vi "quiz3.3.vi"() -> ()   [LabVIEW 2017]
panel:
  out "Tab Control 2":enum32{"Login", "Menu", "Add", "delete"}(tab)
  in  "Ingresar 2":bool
  in  "Contraseña 2":string
  in  "Usuario 2":string
  in  "Delete Button 2":bool
  in  "Add Button 2":bool
  in  "Home Button 2":bool
  out "Cusuario 2":string
  in  "Previous Button 3":bool
  in  "AddContraseña 2":string
  in  "AddUsuario 2":string
  in  "Agregar 2":bool
  out "Agregado 2":bool
  in  "Cancel Button 2":bool
  in  "DeleteUsuario 3":string
  in  "Previous Button 4":bool
  out "text 2":string
  out "Tab Control":enum32{"Login", "Menu", "Add", "delete"}(tab)
  in  "Ingresar":bool
  in  "Contraseña":string
  in  "Usuario":string
  in  "Delete Button":bool
  in  "Add Button":bool
  in  "Home Button":bool
  out "Cusuario":string
  in  "Previous Button":bool
  in  "AddContraseña":string
  in  "AddUsuario":string
  in  "Agregar":bool
  out "Agregado":bool
  in  "Cancel Button":bool
  in  "DeleteUsuario":string
  in  "Previous Button 2":bool
  out "text":string
  # "USTED INGRESO CON EL USUARIO"
  # "USTED INGRESO CON EL USUARIO"
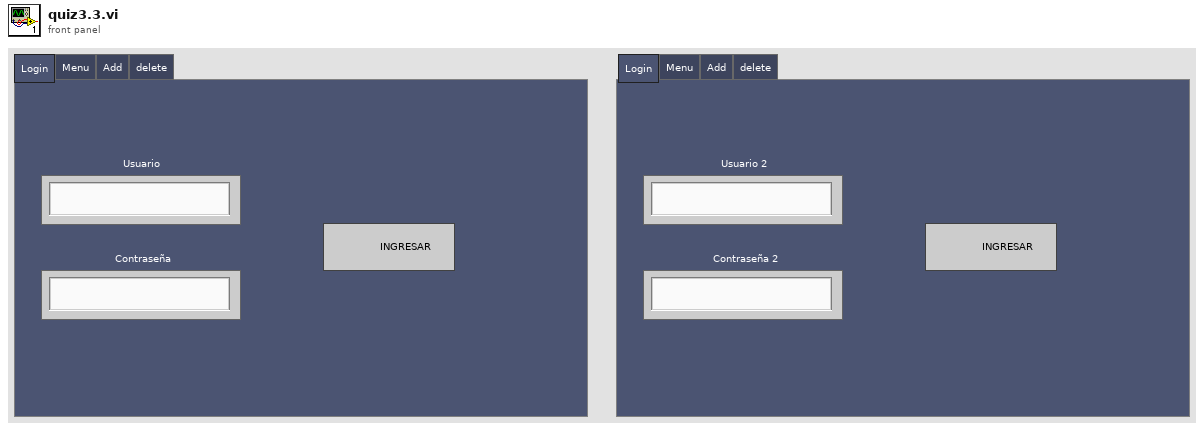
[diagram p1: front panel]
types:
  T1 = enum16{"open", "replace", "create", "open or create", "replace or create", "replace or create with confirmation"}
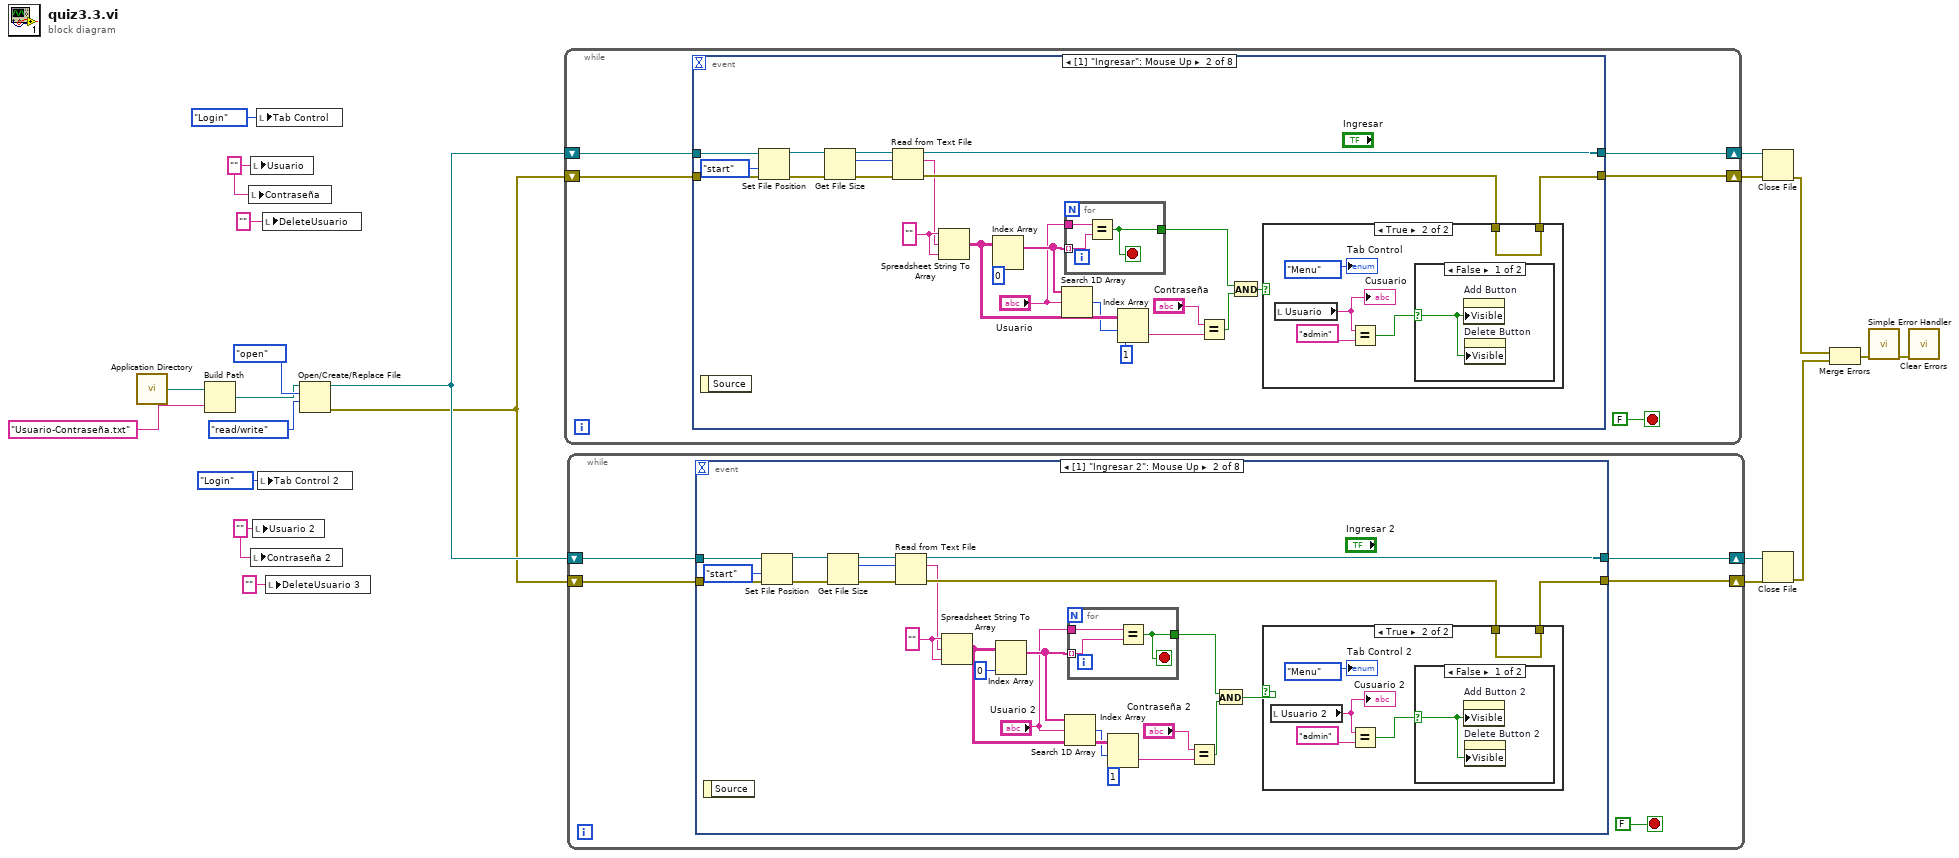
[diagram p0: block diagram]
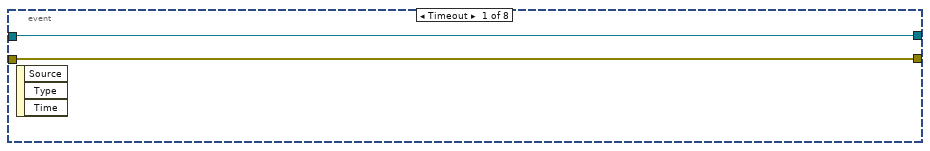
[diagram p2: hidden frame]
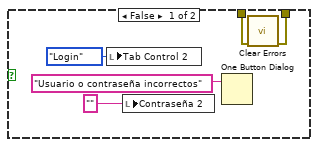
[diagram p3: hidden frame]
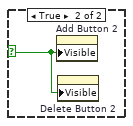
[diagram p4: hidden frame]
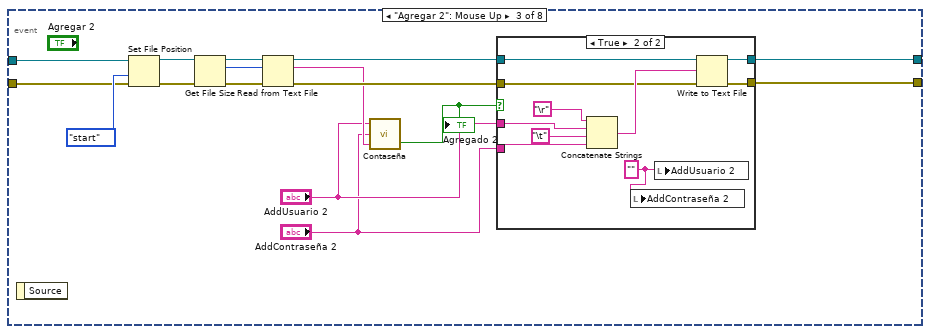
[diagram p5: hidden frame]
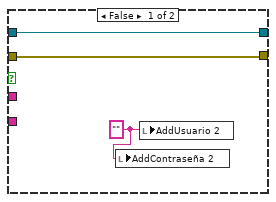
[diagram p6: hidden frame]
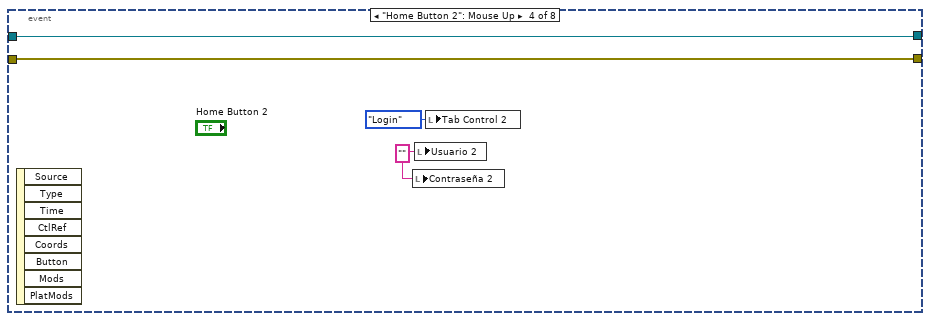
[diagram p7: hidden frame]
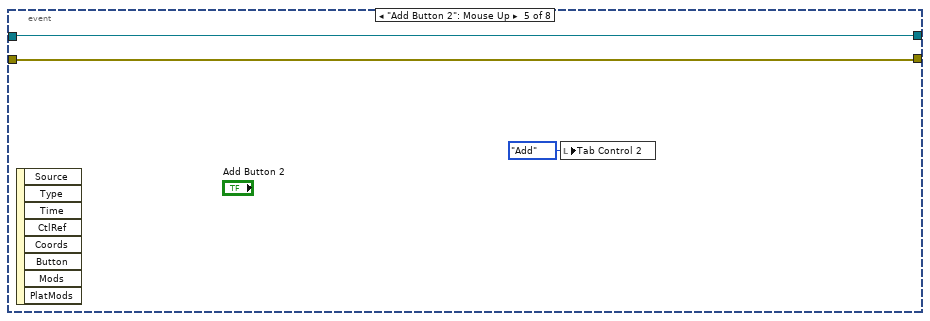
[diagram p8: hidden frame]
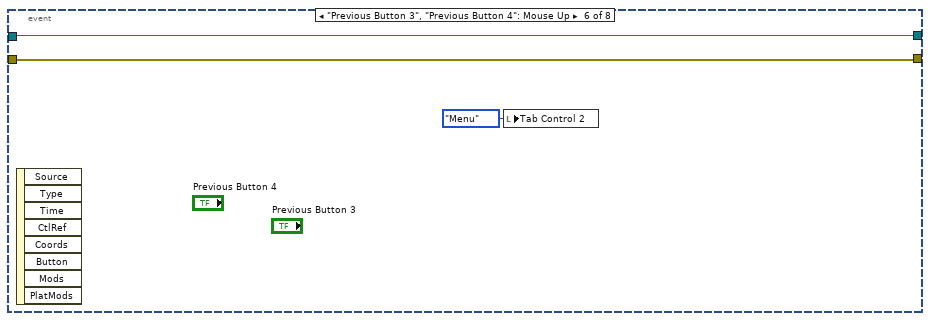
[diagram p9: hidden frame]
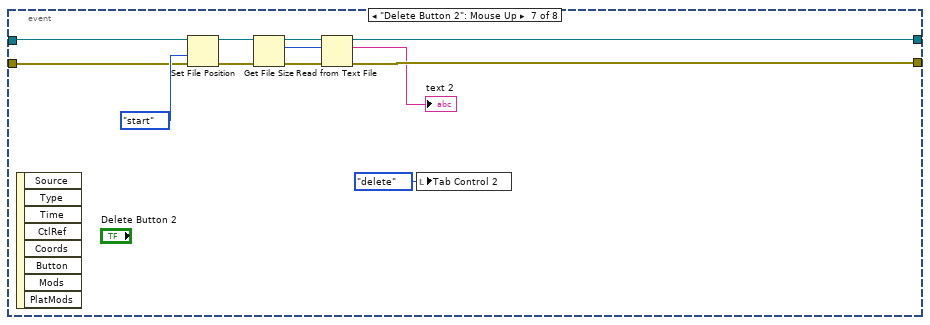
[diagram p10: hidden frame]
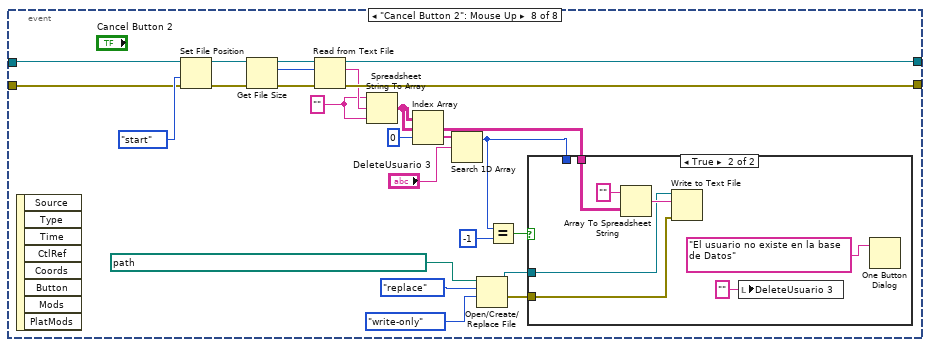
[diagram p11: hidden frame]
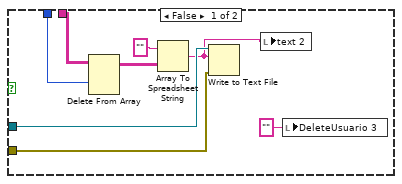
[diagram p12: hidden frame]
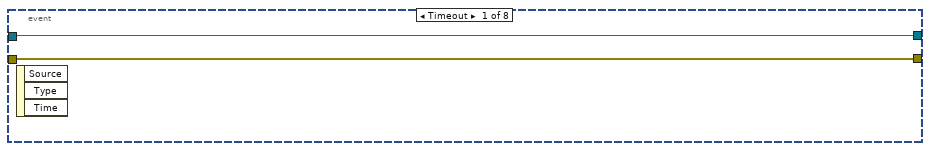
[diagram p13: hidden frame]
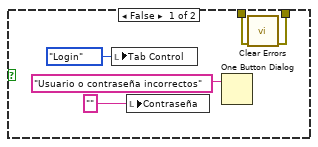
[diagram p14: hidden frame]
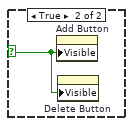
[diagram p15: hidden frame]
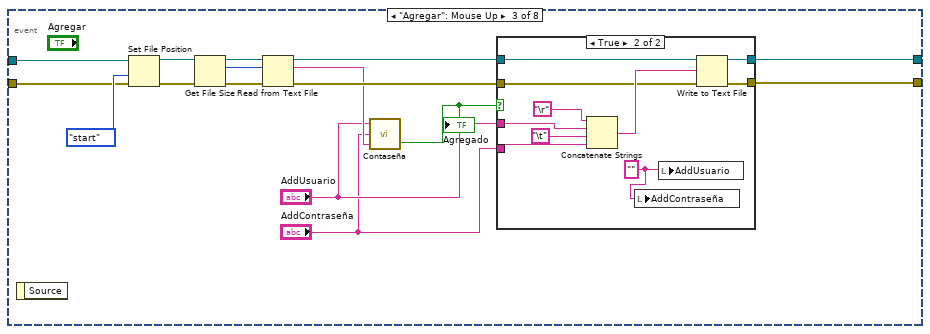
[diagram p16: hidden frame]
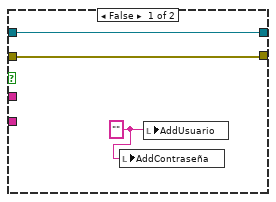
[diagram p17: hidden frame]
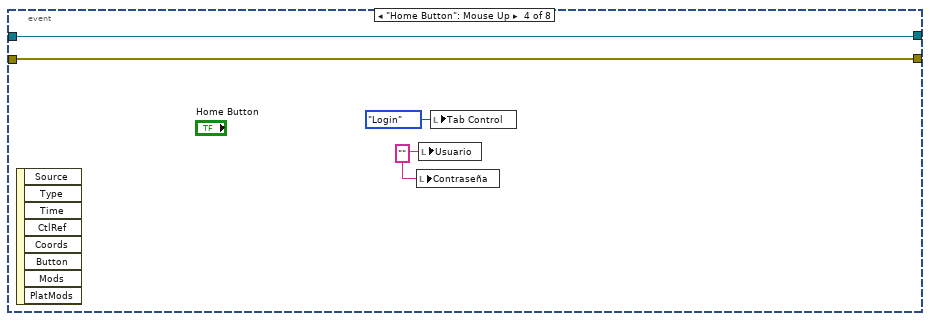
[diagram p18: hidden frame]
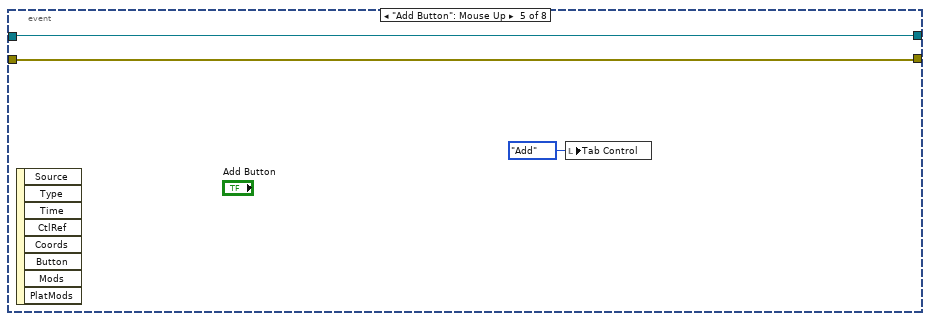
[diagram p19: hidden frame]
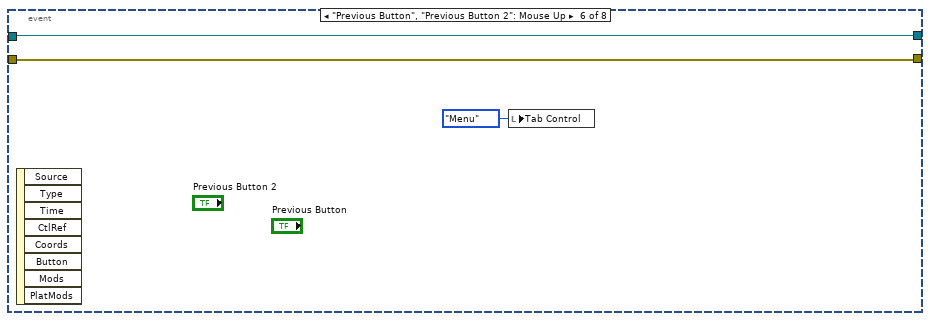
[diagram p20: hidden frame]
diagram:
  w1 = "" ("Usuario")
  w14 = "" ("Usuario")
  n1 = call <vilib>:"Application Directory.vi"() -> ("Application Directory"=w21:path)
  n2 = Build Path(base path=w21, name or relative path="Usuario-Contraseña.txt") -> (appended path=w15:path)
  n3 = local write "Contraseña"(w14) -> ()
  n4 = local write "Usuario"(w14) -> ()
  n5 = local write "Contraseña 2"(w1) -> ()
  n6 = local write "Usuario 2"(w1) -> ()
  n7 = local write "Tab Control"(enum32{"Login", "Menu", "Add", "delete"}."Login" ("Tab Control")) -> ()
  n8 = local write "Tab Control 2"(enum32{"Login", "Menu", "Add", "delete"}."Login" ("Tab Control")) -> ()
  n9 = local write "DeleteUsuario"("" ("DeleteUsuario 2")) -> ()
  n10 = local write "DeleteUsuario 3"("" ("DeleteUsuario 2")) -> ()
  n11 = Open/Create/Replace File(file path (use dialog)=w15, operation (0:open)=T1."open", access (0:read/write)=enum16{"read/write", "read-only", "write-only"}."read/write") -> (refnum out=w5:refnum<file>, error out=w4:errorcluster)  [unwired: 3 in, 1 out]
  n12 = while {
    shift-right: [w23] -> w11
    shift-left: w5 -> [w24]
    shift-right: [w22] -> w16
    shift-left: w4 -> [w25]
    stop <- FALSE stop-if-true
    n13 = event shown="[1] \"Ingresar\": Mouse Up" {
      selector: _ -> [_ _ _ _ _ _ _ _]
      dyn-events: _ -> [_ _ _ _ _ _ _ _]
      timeout: _ -> [_ _ _ _ _ _ _ _]
      tunnel: w25 -> [w27 w52 w71 w98 w102 w105 w109 w136]
      tunnel: [w28 w47 w83 w99 w103 w106 w110 w132] -> w23
      tunnel: [w27 w44 w82 w98 w102 w105 w108 w131] -> w22
      tunnel: w24 -> [w28 w46 w72 w99 w103 w106 w111 w135]
      event Timeout {
        n14 = event-data() -> ()  [unwired: 1 in, 3 out]
      }
      event "Ingresar": Mouse Up {
        w40 = "" ("format string")
        n15 = event-data() -> ()  [unwired: 1 in, 1 out]
        n16 = Set File Position(refnum=w46, from (0:start)=enum16{"start", "end", "current"}."start", error in=w52) -> (refnum out=w50:refnum<file>, error out=w51:errorcluster)  [unwired: 1 in]
        n17 = Get File Size(file=w50, error in=w51) -> (refnum out=w42:refnum<file>, size (in bytes)=w49:i64, 0:w48:errorcluster)
        n18 = Read from Text File(file (use dialog)=w42, count=w49, error in=w48) -> (refnum out=w47:refnum<file>, text=w39:string, error out=w45:errorcluster)  [unwired: 1 in, 1 out]
        n19 = Spreadsheet String To Array(format string=w40, spreadsheet string=w39, array type (2D Dbl)=w40) -> (array=w35:string[][])  [unwired: 1 in]
        n20 = Index Array(array=w35, index (col)=0 ("index")) -> (element=w37:string[])  [unwired: 1 in]
        n21 = Search 1D Array(1D array=w37, element="Usuario") -> (index of element=w32:i32)  [unwired: 1 in]
        n22 = for {
          tunnel: "Usuario" -> [w55]
          tunnel: [w54] -> w38
          tunnel: w37 -> [w53] mode=indexing
          stop <- w54 stop-if-true
          n23 = Equal?(x=w55, y=w53) -> (x = y?=w54:bool)
        }
        n24 = Index Array(array=w35, index (row)=w32, index (col)=1 ("index")) -> (element=w30:string)
        n25 = Equal?(x="Contraseña", y=w30) -> (x = y?=w34:bool)
        n26 = And(x=w38, y=w34) -> (x .and. y?=w41:bool)
        n27 = case shown="True" w41 {
          tunnel: [w58 w65] -> w44
          tunnel: w45 -> [w57 w65]
          frame False {
            n28 = local write "Tab Control"(enum32{"Login", "Menu", "Add", "delete"}."Login" ("Tab Control")) -> ()
            n29 = local write "Contraseña"("" ("Usuario")) -> ()
            n30 = One Button Dialog(message="Usuario o contraseña incorrectos") -> ()  [unwired: 1 in, 1 out]
            n31 = call <vilib>:"Clear Errors.vi"("error in (no error)"=w57) -> ("error out"=w58:errorcluster)  [unwired: 5 in, 1 out]
          }
          frame True {
            n32 = local read "Usuario"() -> (w63:string)
            "Cusuario" <- w63
            n33 = Equal?(x=w63, y="admin") -> (x = y?=w64:bool)
            n34 = case shown="False" w64 {
              selector: w64 -> [w66 w67]
              frame False {
                n35 = property on="Add Button" class="Bool (strict)"("Visible"=w66) -> ()  [unwired: 2 in, 2 out]
                n36 = property on="Delete Button" class="Bool (strict)"("Visible"=w66) -> ()  [unwired: 2 in, 2 out]
              }
              frame True {
                n37 = property on="Add Button" class="Bool (strict)"("Visible"=w67) -> ()  [unwired: 2 in, 2 out]
                n38 = property on="Delete Button" class="Bool (strict)"("Visible"=w67) -> ()  [unwired: 2 in, 2 out]
              }
            }
            "Tab Control" <- enum32{"Login", "Menu", "Add", "delete"}."Menu" ("Tab Control")
          }
        }
      }
      event "Agregar": Mouse Up {
        n39 = event-data() -> ()  [unwired: 1 in, 1 out]
        n40 = Set File Position(refnum=w72, from (0:start)=enum16{"start", "end", "current"}."start", error in=w71) -> (refnum out=w79:refnum<file>, error out=w80:errorcluster)  [unwired: 1 in]
        n41 = Get File Size(file=w79, error in=w80) -> (refnum out=w76:refnum<file>, size (in bytes)=w78:i64, 0:w77:errorcluster)
        n42 = Read from Text File(file (use dialog)=w76, count=w78, error in=w77) -> (refnum out=w74:refnum<file>, text=w70:string, error out=w73:errorcluster)  [unwired: 1 in, 1 out]
        n43 = call "Contaseña.vi"("spreadsheet string"=w70, "AddContraseña"="AddContraseña", "addUsuario"="AddUsuario") -> ("result"=w81:bool)  [unwired: 1 out]
        "Agregado" <- w81
        n44 = case shown="True" w81 {
          tunnel: [w86 w96] -> w83
          tunnel: [w85 w95] -> w82
          tunnel: w74 -> [w86 w91]
          tunnel: w73 -> [w85 w90]
          tunnel: "AddUsuario" -> [_ w89]
          tunnel: "AddContraseña" -> [_ w88]
          frame False {
            w84 = "" ("Usuario")
            n45 = local write "AddContraseña"(w84) -> ()
            n46 = local write "AddUsuario"(w84) -> ()
          }
          frame True {
            w87 = "" ("Usuario")
            n47 = Concatenate Strings("\r", w89, "\t", w88) -> (w94:string)
            n48 = local write "AddContraseña"(w87) -> ()
            n49 = local write "AddUsuario"(w87) -> ()
            n50 = Write to Text File(file (use dialog)=w91, text=w94, error in=w90) -> (refnum out=w96:refnum<file>, error out=w95:errorcluster)  [unwired: 1 in, 1 out]
          }
        }
      }
      event "Home Button": Mouse Up {
        w100 = "" ("Usuario")
        n51 = event-data() -> ()  [unwired: 1 in, 8 out]
        n52 = local write "Contraseña"(w100) -> ()
        n53 = local write "Usuario"(w100) -> ()
        n54 = local write "Tab Control"(enum32{"Login", "Menu", "Add", "delete"}."Login" ("Tab Control")) -> ()
      }
      event "Add Button": Mouse Up {
        n55 = event-data() -> ()  [unwired: 1 in, 8 out]
        n56 = local write "Tab Control"(enum32{"Login", "Menu", "Add", "delete"}."Add" ("Tab Control")) -> ()
      }
      event "Previous Button", "Previous Button 2": Mouse Up {
        n57 = event-data() -> ()  [unwired: 1 in, 8 out]
        n58 = local write "Tab Control"(enum32{"Login", "Menu", "Add", "delete"}."Menu" ("Tab Control")) -> ()
      }
      event "Delete Button": Mouse Up {
        n59 = event-data() -> ()  [unwired: 1 in, 8 out]
        n60 = Set File Position(refnum=w111, from (0:start)=enum16{"start", "end", "current"}."start", error in=w109) -> (refnum out=w116:refnum<file>, error out=w117:errorcluster)  [unwired: 1 in]
        n61 = Get File Size(file=w116, error in=w117) -> (refnum out=w113:refnum<file>, size (in bytes)=w115:i64, 0:w114:errorcluster)
        n62 = Read from Text File(file (use dialog)=w113, count=w115, error in=w114) -> (refnum out=w110:refnum<file>, text=→"text":string, error out=w108:errorcluster)  [unwired: 1 in, 1 out]
        n63 = local write "Tab Control"(enum32{"Login", "Menu", "Add", "delete"}."delete" ("Tab Control")) -> ()
      }
      event "Cancel Button": Mouse Up {
        w128 = "" ("format string")
        n64 = event-data() -> ()  [unwired: 1 in, 8 out]
        n65 = Set File Position(refnum=w135, from (0:start)=enum16{"start", "end", "current"}."start", error in=w136) -> (refnum out=w141:refnum<file>, error out=w142:errorcluster)  [unwired: 1 in]
        n66 = Get File Size(file=w141, error in=w142) -> (refnum out=w138:refnum<file>, size (in bytes)=w140:i64, 0:w139:errorcluster)
        n67 = Read from Text File(file (use dialog)=w138, count=w140, error in=w139) -> (refnum out=w132:refnum<file>, text=w129:string, error out=w131:errorcluster)  [unwired: 1 in, 1 out]
        n68 = Spreadsheet String To Array(format string=w128, spreadsheet string=w129, array type (2D Dbl)=w128) -> (array=w124:string[][])  [unwired: 1 in]
        n69 = Index Array(array=w124, index (col)=0 ("disabled index (col)")) -> (element=w126:string[])  [unwired: 1 in]
        n70 = Search 1D Array(1D array=w126, element="DeleteUsuario") -> (index of element=w120:i32)  [unwired: 1 in]
        n71 = Open/Create/Replace File(file path (use dialog)=path "D:/2019-1/Programacion 2/quiz 3/Usuario-Contraseña.txt", operation (0:open)=T1."replace", access (0:read/write)=enum16{"read/write", "read-only", "write-only"}."write-only") -> (refnum out=w123:refnum<file>, error out=w122:errorcluster)  [unwired: 3 in, 1 out]
        n72 = Equal?(x=w120, y=-1) -> (x = y?=w121:bool)
        n73 = case shown="True" w121 {
          tunnel: w124 -> [w150 w153]
          tunnel: w120 -> [w149 _]
          tunnel: w123 -> [w147 w152]
          tunnel: w122 -> [w146 w151]
          frame False {
            n74 = Delete From Array(array=w150, index (row)=w149) -> (array with subset deleted=w148:string[][])  [unwired: 2 in, 1 out]
            n75 = Array To Spreadsheet String(array=w148, 3:"" ("format string")) -> (spreadsheet string=w144:string)  [unwired: 1 in]
            n76 = Write to Text File(file (use dialog)=w147, text=w144, error in=w146) -> ()  [unwired: 1 in, 3 out]
            n77 = local write "text"(w144) -> ()
            n78 = local write "DeleteUsuario"("" ("DeleteUsuario 2")) -> ()
          }
          frame True {
            n79 = Array To Spreadsheet String(array=w153, 3:"" ("format string")) -> (spreadsheet string=w155:string)  [unwired: 1 in]
            n80 = Write to Text File(file (use dialog)=w152, text=w155, error in=w151) -> ()  [unwired: 1 in, 3 out]
            n81 = local write "DeleteUsuario"("" ("DeleteUsuario 2")) -> ()
            n82 = One Button Dialog(message="El usuario no existe en la base de Datos") -> ()  [unwired: 1 in, 1 out]
          }
        }
      }
    }
  }
  n83 = while {
    shift-right: [w159] -> w6
    shift-left: w5 -> [w160]
    shift-right: [w158] -> w7
    shift-left: w4 -> [w161]
    stop <- FALSE stop-if-true
    n84 = event shown="[1] \"Ingresar 2\": Mouse Up" {
      selector: _ -> [_ _ _ _ _ _ _ _]
      dyn-events: _ -> [_ _ _ _ _ _ _ _]
      timeout: _ -> [_ _ _ _ _ _ _ _]
      tunnel: w161 -> [w163 w188 w207 w234 w238 w241 w245 w272]
      tunnel: [w164 w183 w219 w235 w239 w242 w246 w268] -> w159
      tunnel: [w163 w180 w218 w234 w238 w241 w244 w267] -> w158
      tunnel: w160 -> [w164 w182 w208 w235 w239 w242 w247 w271]
      event Timeout {
        n85 = event-data() -> ()  [unwired: 1 in, 3 out]
      }
      event "Ingresar 2": Mouse Up {
        w176 = "" ("format string")
        n86 = event-data() -> ()  [unwired: 1 in, 1 out]
        n87 = Set File Position(refnum=w182, from (0:start)=enum16{"start", "end", "current"}."start", error in=w188) -> (refnum out=w186:refnum<file>, error out=w187:errorcluster)  [unwired: 1 in]
        n88 = Get File Size(file=w186, error in=w187) -> (refnum out=w178:refnum<file>, size (in bytes)=w185:i64, 0:w184:errorcluster)
        n89 = Read from Text File(file (use dialog)=w178, count=w185, error in=w184) -> (refnum out=w183:refnum<file>, text=w175:string, error out=w181:errorcluster)  [unwired: 1 in, 1 out]
        n90 = Spreadsheet String To Array(format string=w176, spreadsheet string=w175, array type (2D Dbl)=w176) -> (array=w171:string[][])  [unwired: 1 in]
        n91 = Index Array(array=w171, index (col)=0 ("index")) -> (element=w173:string[])  [unwired: 1 in]
        n92 = Search 1D Array(1D array=w173, element="Usuario 2") -> (index of element=w168:i32)  [unwired: 1 in]
        n93 = for {
          tunnel: "Usuario 2" -> [w191]
          tunnel: [w190] -> w174
          tunnel: w173 -> [w189] mode=indexing
          stop <- w190 stop-if-true
          n94 = Equal?(x=w191, y=w189) -> (x = y?=w190:bool)
        }
        n95 = Index Array(array=w171, index (row)=w168, index (col)=1 ("index")) -> (element=w166:string)
        n96 = Equal?(x="Contraseña 2", y=w166) -> (x = y?=w170:bool)
        n97 = And(x=w174, y=w170) -> (x .and. y?=w177:bool)
        n98 = case shown="True" w177 {
          tunnel: [w194 w201] -> w180
          tunnel: w181 -> [w193 w201]
          frame False {
            n99 = local write "Tab Control 2"(enum32{"Login", "Menu", "Add", "delete"}."Login" ("Tab Control")) -> ()
            n100 = local write "Contraseña 2"("" ("Usuario")) -> ()
            n101 = One Button Dialog(message="Usuario o contraseña incorrectos") -> ()  [unwired: 1 in, 1 out]
            n102 = call <vilib>:"Clear Errors.vi"("error in (no error)"=w193) -> ("error out"=w194:errorcluster)  [unwired: 5 in, 1 out]
          }
          frame True {
            n103 = local read "Usuario 2"() -> (w199:string)
            "Cusuario 2" <- w199
            n104 = Equal?(x=w199, y="admin") -> (x = y?=w200:bool)
            n105 = case shown="False" w200 {
              selector: w200 -> [w202 w203]
              frame False {
                n106 = property on="Add Button 2" class="Bool (strict)"("Visible"=w202) -> ()  [unwired: 2 in, 2 out]
                n107 = property on="Delete Button 2" class="Bool (strict)"("Visible"=w202) -> ()  [unwired: 2 in, 2 out]
              }
              frame True {
                n108 = property on="Add Button 2" class="Bool (strict)"("Visible"=w203) -> ()  [unwired: 2 in, 2 out]
                n109 = property on="Delete Button 2" class="Bool (strict)"("Visible"=w203) -> ()  [unwired: 2 in, 2 out]
              }
            }
            "Tab Control 2" <- enum32{"Login", "Menu", "Add", "delete"}."Menu" ("Tab Control")
          }
        }
      }
      event "Agregar 2": Mouse Up {
        n110 = event-data() -> ()  [unwired: 1 in, 1 out]
        n111 = Set File Position(refnum=w208, from (0:start)=enum16{"start", "end", "current"}."start", error in=w207) -> (refnum out=w215:refnum<file>, error out=w216:errorcluster)  [unwired: 1 in]
        n112 = Get File Size(file=w215, error in=w216) -> (refnum out=w212:refnum<file>, size (in bytes)=w214:i64, 0:w213:errorcluster)
        n113 = Read from Text File(file (use dialog)=w212, count=w214, error in=w213) -> (refnum out=w210:refnum<file>, text=w206:string, error out=w209:errorcluster)  [unwired: 1 in, 1 out]
        n114 = call "Contaseña.vi"("spreadsheet string"=w206, "AddContraseña"="AddContraseña 2", "addUsuario"="AddUsuario 2") -> ("result"=w217:bool)  [unwired: 1 out]
        "Agregado 2" <- w217
        n115 = case shown="True" w217 {
          tunnel: [w222 w232] -> w219
          tunnel: [w221 w231] -> w218
          tunnel: w210 -> [w222 w227]
          tunnel: w209 -> [w221 w226]
          tunnel: "AddUsuario 2" -> [_ w225]
          tunnel: "AddContraseña 2" -> [_ w224]
          frame False {
            w220 = "" ("Usuario")
            n116 = local write "AddContraseña 2"(w220) -> ()
            n117 = local write "AddUsuario 2"(w220) -> ()
          }
          frame True {
            w223 = "" ("Usuario")
            n118 = Concatenate Strings("\r", w225, "\t", w224) -> (w230:string)
            n119 = local write "AddContraseña 2"(w223) -> ()
            n120 = local write "AddUsuario 2"(w223) -> ()
            n121 = Write to Text File(file (use dialog)=w227, text=w230, error in=w226) -> (refnum out=w232:refnum<file>, error out=w231:errorcluster)  [unwired: 1 in, 1 out]
          }
        }
      }
      event "Home Button 2": Mouse Up {
        w236 = "" ("Usuario")
        n122 = event-data() -> ()  [unwired: 1 in, 8 out]
        n123 = local write "Contraseña 2"(w236) -> ()
        n124 = local write "Usuario 2"(w236) -> ()
        n125 = local write "Tab Control 2"(enum32{"Login", "Menu", "Add", "delete"}."Login" ("Tab Control")) -> ()
      }
      event "Add Button 2": Mouse Up {
        n126 = event-data() -> ()  [unwired: 1 in, 8 out]
        n127 = local write "Tab Control 2"(enum32{"Login", "Menu", "Add", "delete"}."Add" ("Tab Control")) -> ()
      }
      event "Previous Button 3", "Previous Button 4": Mouse Up {
        n128 = event-data() -> ()  [unwired: 1 in, 8 out]
        n129 = local write "Tab Control 2"(enum32{"Login", "Menu", "Add", "delete"}."Menu" ("Tab Control")) -> ()
      }
      event "Delete Button 2": Mouse Up {
        n130 = event-data() -> ()  [unwired: 1 in, 8 out]
        n131 = Set File Position(refnum=w247, from (0:start)=enum16{"start", "end", "current"}."start", error in=w245) -> (refnum out=w252:refnum<file>, error out=w253:errorcluster)  [unwired: 1 in]
        n132 = Get File Size(file=w252, error in=w253) -> (refnum out=w249:refnum<file>, size (in bytes)=w251:i64, 0:w250:errorcluster)
        n133 = Read from Text File(file (use dialog)=w249, count=w251, error in=w250) -> (refnum out=w246:refnum<file>, text=→"text 2":string, error out=w244:errorcluster)  [unwired: 1 in, 1 out]
        n134 = local write "Tab Control 2"(enum32{"Login", "Menu", "Add", "delete"}."delete" ("Tab Control")) -> ()
      }
      event "Cancel Button 2": Mouse Up {
        w264 = "" ("format string")
        n135 = event-data() -> ()  [unwired: 1 in, 8 out]
        n136 = Set File Position(refnum=w271, from (0:start)=enum16{"start", "end", "current"}."start", error in=w272) -> (refnum out=w277:refnum<file>, error out=w278:errorcluster)  [unwired: 1 in]
        n137 = Get File Size(file=w277, error in=w278) -> (refnum out=w274:refnum<file>, size (in bytes)=w276:i64, 0:w275:errorcluster)
        n138 = Read from Text File(file (use dialog)=w274, count=w276, error in=w275) -> (refnum out=w268:refnum<file>, text=w265:string, error out=w267:errorcluster)  [unwired: 1 in, 1 out]
        n139 = Spreadsheet String To Array(format string=w264, spreadsheet string=w265, array type (2D Dbl)=w264) -> (array=w260:string[][])  [unwired: 1 in]
        n140 = Index Array(array=w260, index (col)=0 ("disabled index (col)")) -> (element=w262:string[])  [unwired: 1 in]
        n141 = Search 1D Array(1D array=w262, element="DeleteUsuario 3") -> (index of element=w256:i32)  [unwired: 1 in]
        n142 = Open/Create/Replace File(file path (use dialog)=path "D:/2019-1/Programacion 2/quiz 3/Usuario-Contraseña.txt", operation (0:open)=T1."replace", access (0:read/write)=enum16{"read/write", "read-only", "write-only"}."write-only") -> (refnum out=w259:refnum<file>, error out=w258:errorcluster)  [unwired: 3 in, 1 out]
        n143 = Equal?(x=w256, y=-1) -> (x = y?=w257:bool)
        n144 = case shown="True" w257 {
          tunnel: w260 -> [w286 w289]
          tunnel: w256 -> [w285 _]
          tunnel: w259 -> [w283 w288]
          tunnel: w258 -> [w282 w287]
          frame False {
            n145 = Delete From Array(array=w286, index (row)=w285) -> (array with subset deleted=w284:string[][])  [unwired: 2 in, 1 out]
            n146 = Array To Spreadsheet String(array=w284, 3:"" ("format string")) -> (spreadsheet string=w280:string)  [unwired: 1 in]
            n147 = Write to Text File(file (use dialog)=w283, text=w280, error in=w282) -> ()  [unwired: 1 in, 3 out]
            n148 = local write "text 2"(w280) -> ()
            n149 = local write "DeleteUsuario 3"("" ("DeleteUsuario 2")) -> ()
          }
          frame True {
            n150 = Array To Spreadsheet String(array=w289, 3:"" ("format string")) -> (spreadsheet string=w291:string)  [unwired: 1 in]
            n151 = Write to Text File(file (use dialog)=w288, text=w291, error in=w287) -> ()  [unwired: 1 in, 3 out]
            n152 = local write "DeleteUsuario 3"("" ("DeleteUsuario 2")) -> ()
            n153 = One Button Dialog(message="El usuario no existe en la base de Datos") -> ()  [unwired: 1 in, 1 out]
          }
        }
      }
    }
  }
  n154 = Close File(refnum=w11, error in=w16) -> (error out=w9:errorcluster)  [unwired: 1 out]
  n155 = Close File(refnum=w6, error in=w7) -> (error out=w8:errorcluster)  [unwired: 1 out]
  n156 = Merge Errors(w9, w8) -> (w10:errorcluster)
  n157 = call <vilib>:"Simple Error Handler.vi"("error in (no error)"=w10) -> ("error out"=w17:errorcluster)  [unwired: 4 in, 4 out]
  n158 = call <vilib>:"Clear Errors.vi"("error in (no error)"=w17) -> ()  [unwired: 5 in, 2 out]
